vi "判断闰年.vi"(1 "Year":u16) -> (0 "Leap":bool)   [LabVIEW 2011]
doc: "功能：\n\n判断输入年份是否为闰年。\n\n规则：\n\n((year%4==0 && year%100!=0) ||year%400==0)\n\ncsxcs_366创建"
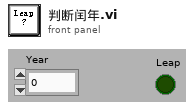
[diagram p1: front panel]
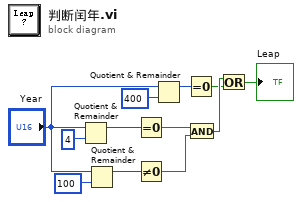
[diagram p0: block diagram]
diagram:
  n1 = Quotient & Remainder(x="Year", y=u16 4) -> (x-y*floor(x/y)=w10:u16)  [unwired: 1 out]
  n2 = Quotient & Remainder(x="Year", y=u16 100) -> (x-y*floor(x/y)=w6:u16)  [unwired: 1 out]
  n3 = Equal To 0?(x=w10) -> (x = 0?=w9:bool)
  n4 = Not Equal To 0?(x=w6) -> (x != 0?=w8:bool)
  n5 = Quotient & Remainder(x="Year", y=u16 400) -> (x-y*floor(x/y)=w3:u16)  [unwired: 1 out]
  n6 = Equal To 0?(x=w3) -> (x = 0?=w2:bool)
  n7 = And(x=w9, y=w8) -> (x .and. y?=w7:bool)
  n8 = Or(x=w7, y=w2) -> (x .or. y?=→"Leap":bool)
